vi "Initialize.vi"(8 "error in":errorcluster, 11 "TSI 3081 Long in":refnum<class "TSI 3081 Long.lvclass">) -> (0 "error out":errorcluster, 3 "TSI 3081 Long out":refnum<class "TSI 3081 Long.lvclass">)   [LabVIEW 2014, in "TSI 3081 Long.lvclass"]
uses:
  TSI 3081 Long.lvclass
  DMA.lvclass/DMA.ctl
  Accessors/Write ri.vi
  Accessors/Write ro.vi
  Accessors/Write Leff.vi
  DMA.lvclass
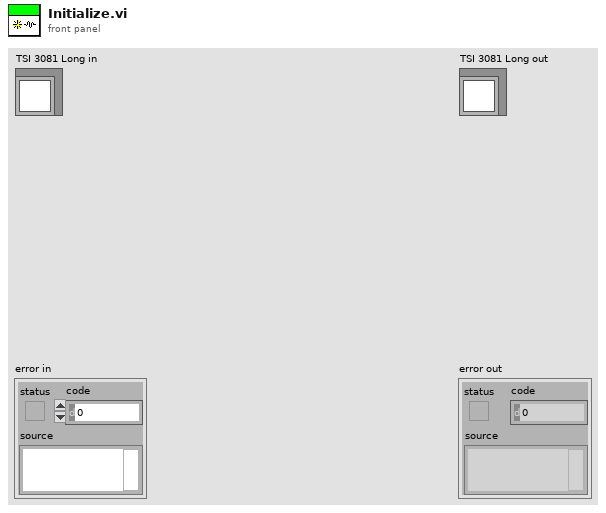
[diagram p1: front panel]
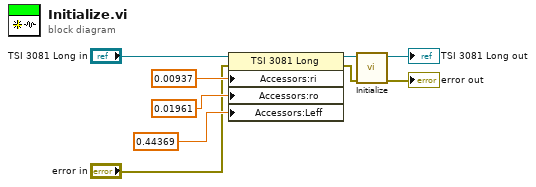
[diagram p0: block diagram]
diagram:
  n1 = property class="TSI 3081 Long"(reference="TSI 3081 Long in", error in="error in", "Accessors:ri"=0.00937 ("ri"), "Accessors:ro"=0.01961 ("ro"), "Accessors:Leff"=0.44369 ("Leff")) -> (reference out=w9:refnum<class "TSI 3081 Long.lvclass">, error out=w5:errorcluster)
  n2 = call-parent "Initialize.vi"("error in"=w5, "DMA in"=w9) -> ("error out"=→"error out":errorcluster, "DMA out"=→"TSI 3081 Long out":refnum<class "TSI 3081 Long.lvclass">)  [unwired: 8 in]
